vi "Main.vi"(10 "JQMHStartup.lvclass":refnum<class "JQMHStartup.lvclass">, 11 "JQMHCore in":refnum<class "JQMHModule.lvclass">) -> ()   [LabVIEW 2024, in "JQMHModule.lvclass"]
uses:
  JQMHModule.lvclass
  JQMHStartup/JQMHStartup.lvclass
  JQMHModule.lvclass/JQMHModule.ctl
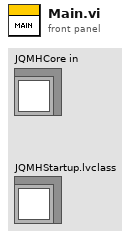
[diagram p1: front panel]
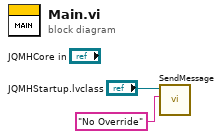
[diagram p0: block diagram]
diagram:
  n1 = call "SendMessage.vi"("Command"="No Override", "JQMHStartup in"="JQMHStartup.lvclass") -> ()  [unwired: 8 in, 2 out]
